vi "TestDllCall.vi"() -> ()   [LabVIEW 2017]
uses:
  D:/Project/Tymphany/HDMI Board_2025-04-15/HDMI Board/LT_UpgradeFlash_Lib/LT_UpgradeFlash_Lib/bin/Debug/LT_UpgradeFlash_Lib.dll
  LT_UpgradeFlash_Lib/bin/Debug/LT_UpgradeFlash_Lib.dll
panel:
  in  "stop":bool
  in  "changeChip":bool
  in  "chipSelection":string="LT6911(UX/UXB/UXC)"
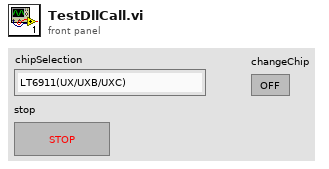
[diagram p1: front panel]
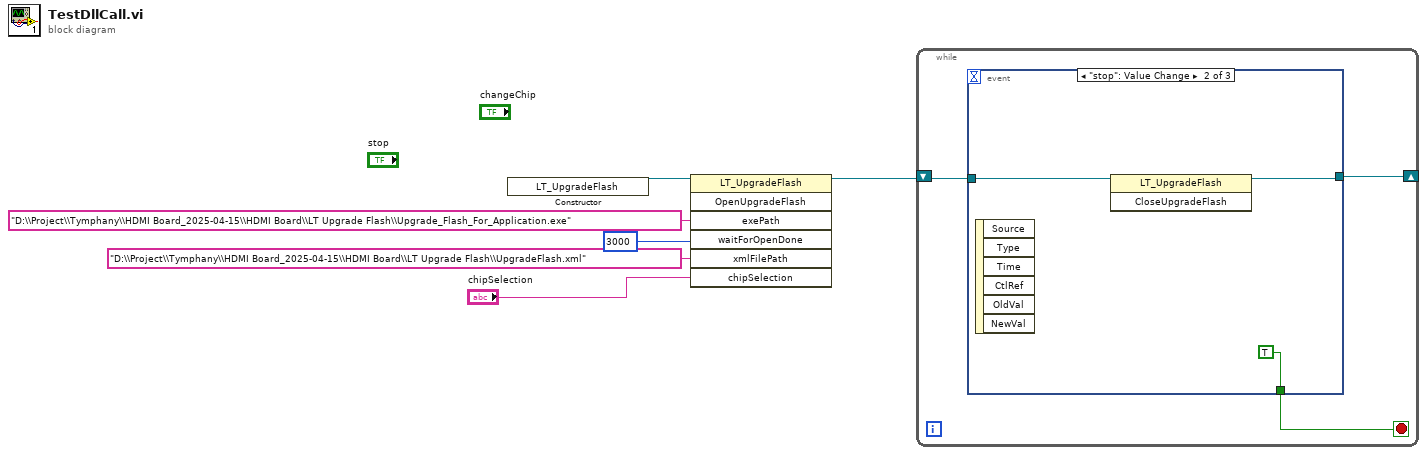
[diagram p0: block diagram]
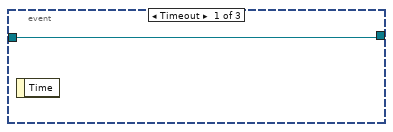
[diagram p2: hidden frame]
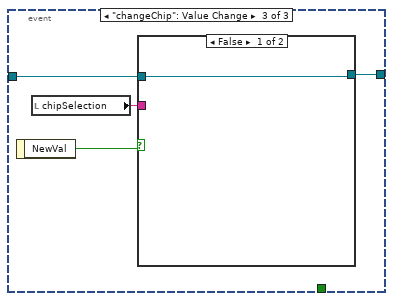
[diagram p3: hidden frame]
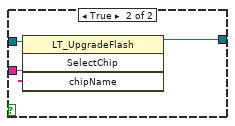
[diagram p4: hidden frame]
diagram:
  n1 = constructor class="LT_UpgradeFlash"() -> (reference out=w6:refnum<k24>)  [unwired: 3 in, 2 out]
  n2 = invoke class="LT_UpgradeFlash" method="OpenUpgradeFlash"(reference=w6, "exePath"="D:\\Project\\Tymphany\\HDMI Board_2025-04-15\\HDMI Board\\LT Upgrade Flash\\Upgrade_Flash_For_Application.exe", "waitForOpenDone"=3000, "xmlFilePath"="D:\\Project\\Tymphany\\HDMI Board_2025-04-15\\HDMI Board\\LT Upgrade Flash\\UpgradeFlash.xml", "chipSelection"="chipSelection") -> (reference out=w1:refnum<k24>)  [unwired: 2 in, 6 out]
  n3 = while {
    shift-right: [w7] -> _
    shift-left: w1 -> [w9]
    stop <- w8 stop-if-true
    n4 = event shown="[1] \"stop\": Value Change" {
      selector: _ -> [_ _ _]
      dyn-events: _ -> [_ _ _]
      timeout: _ -> [_ _ _]
      tunnel: w9 -> [w10 w12 w16]
      tunnel: [_ TRUE _] -> w8
      tunnel: [w10 w11 w14] -> w7
      event Timeout {
        n5 = event-data() -> ()  [unwired: 1 in, 1 out]
      }
      event "stop": Value Change {
        n6 = event-data() -> ()  [unwired: 1 in, 6 out]
        n7 = invoke class="LT_UpgradeFlash" method="CloseUpgradeFlash"(reference=w12) -> (reference out=w11:refnum<k24>)  [unwired: 2 in, 2 out]
      }
      event "changeChip": Value Change {
        n8 = event-data() -> ("NewVal"=w17:bool)  [unwired: 1 in]
        n9 = local read "chipSelection"() -> (w15:string)
        n10 = case shown="False" w17 {
          tunnel: w16 -> [w18 w21]
          tunnel: w15 -> [_ w20]
          tunnel: [w18 w19] -> w14
          frame False {
          }
          frame True {
            n11 = invoke class="LT_UpgradeFlash" method="SelectChip"(reference=w21, "chipName"=w20) -> (reference out=w19:refnum<k24>)  [unwired: 2 in, 3 out]
          }
        }
      }
    }
  }
